vi "Convert to tiff.vi"(7 "downcast to 8-bit? (F)":bool, 8 "error in (no error)":errorcluster, 9 "source file":path, 10 "Destination directory":path, 11 "reference to path":refnum<vi>) -> (0 "error out":errorcluster)   [LabVIEW 2012]
panel:
  out "Path":path
  out "Slide":sgl(slide) scale=0.0..1.0
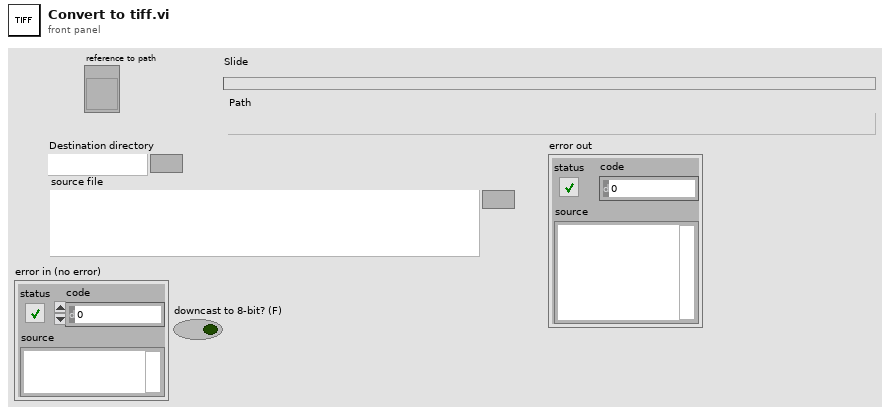
[diagram p1: front panel]
types:
  T1 = typedef "Image Type" = u32
  T2 = typedef "IMAQ Image.ctl" = refnum<image>
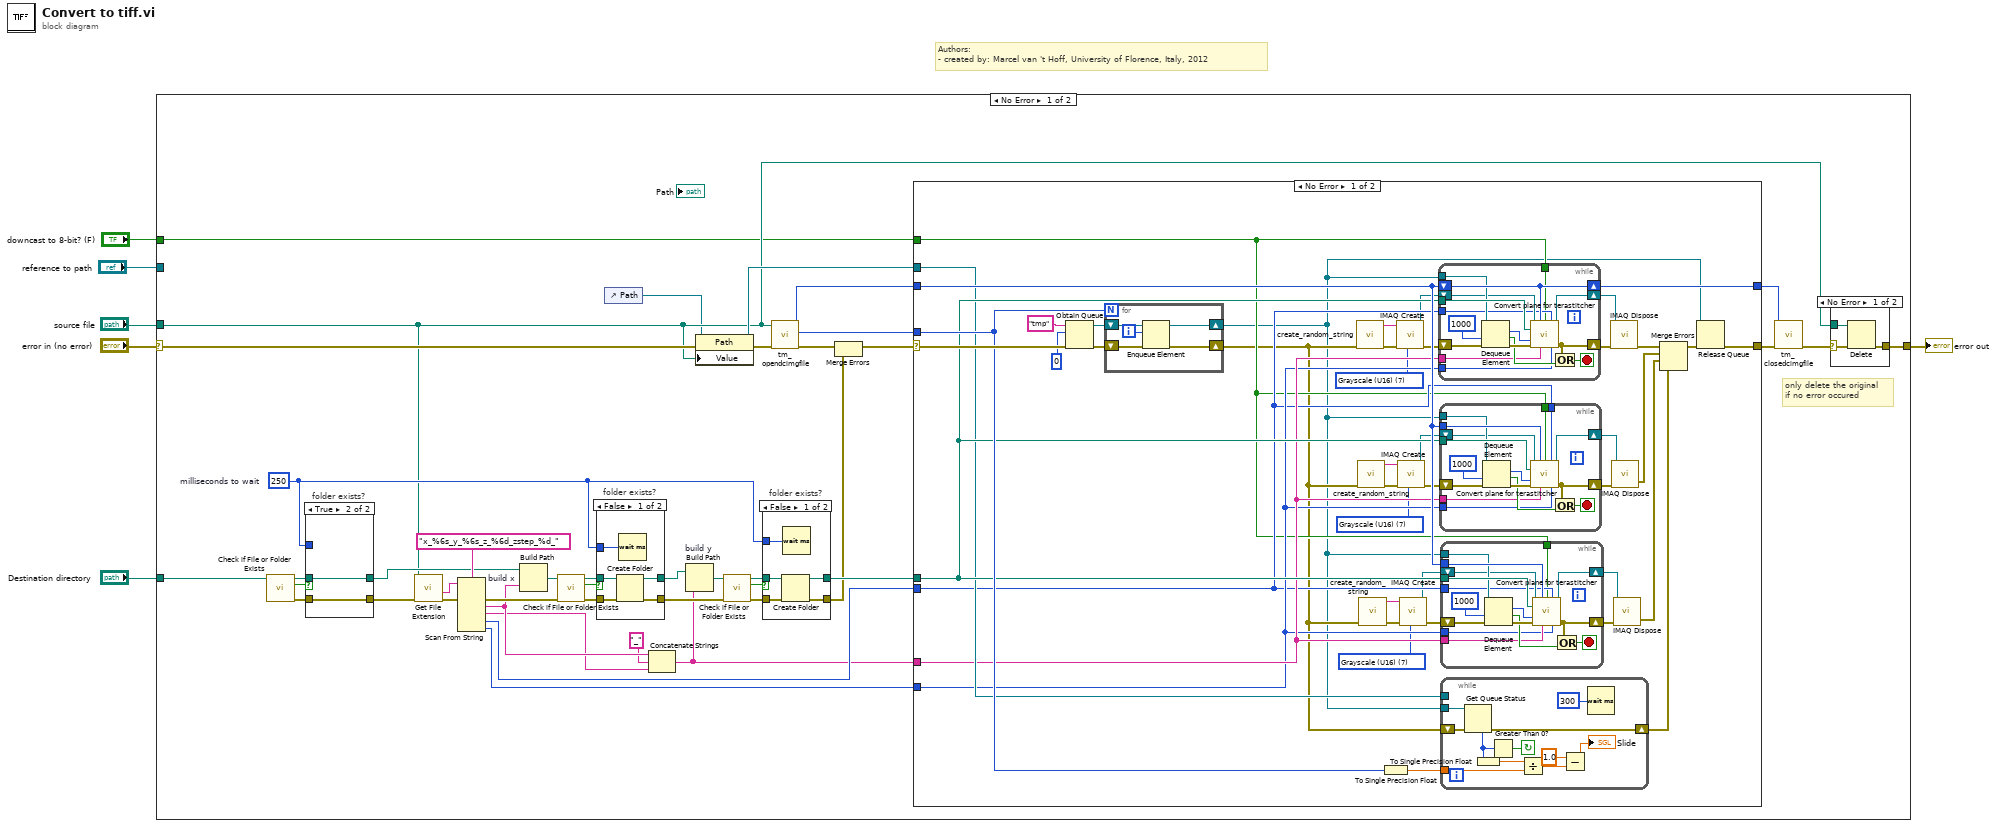
[diagram p0: block diagram]
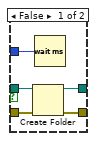
[diagram p5: hidden frame]
diagram:
  # "Authors: \n- created by: Marcel van 't Hoff, University of Florence, Italy, 2012"
  n1 = case shown="No Error" "error in (no error)" {
    selector: "error in (no error)" -> [w49 w185]
    tunnel: [w11 w185] -> w3
    tunnel: "source file" -> [w10 _]
    tunnel: "Destination directory" -> [w43 _]
    tunnel: "reference to path" -> [_ _]
    tunnel: "downcast to 8-bit? (F)" -> [w9 _]
    frame No Error {
      w12 = u32 250  # milliseconds to wait
      # "only delete the original\nif no error occured"
      n2 = call <vilib>:"Check if File or Folder Exists.vi"("path"=w43) -> ("error out"=w40:errorcluster, "file or folder exists?"=w41:bool, "dup path"=w42:path)  [unwired: 8 in]
      n3 = case "folder exists?" shown="True" w41 {
        tunnel: [w72 w74] -> w22
        tunnel: w42 -> [w71 w74]
        tunnel: w40 -> [w70 w73]
        tunnel: [w69 w73] -> w35
        tunnel: w12 -> [w68 _]
        frame False {
          n4 = Create Folder(path (use dialog)=w71, error in=w70) -> (created path=w72:path, error out=w69:errorcluster)  [unwired: 1 in, 1 out]
          n5 = Wait (ms)(milliseconds to wait=w68) -> ()  [unwired: 1 out]
        }
        frame True {
        }
      }
      n6 = call <vilib>:"Get File Extension.vi"("error in (no error)"=w35, "file"=w10) -> ("error out"=w36:errorcluster, "filename without extension"=w37:string)  [unwired: 6 in, 2 out]
      n7 = Scan From String(format string="x_%6s_y_%6s_z_%6d_zstep_%d_", input string=w37, error in=w36) -> (error out=w31:errorcluster, output 1=w21:string, output 2=w19:string, output 3=w17:i32, output 4=w18:i32)  [unwired: 5 in, 2 out]
      n8 = Build Path "build x"(base path=w22, name or relative path=w21) -> (appended path=w30:path)
      n9 = call <vilib>:"Check if File or Folder Exists.vi"("error in (no error)"=w31, "path"=w30) -> ("error out"=w34:errorcluster, "file or folder exists?"=w33:bool, "dup path"=w32:path)  [unwired: 7 in]
      n10 = case "folder exists?" shown="False" w33 {
        tunnel: [w65 w67] -> w25
        tunnel: w32 -> [w64 w67]
        tunnel: w34 -> [w63 w66]
        tunnel: [w62 w66] -> w24
        tunnel: w12 -> [w61 _]
        frame False {
          n11 = Create Folder(path (use dialog)=w64, error in=w63) -> (created path=w65:path, error out=w62:errorcluster)  [unwired: 1 in, 1 out]
          n12 = Wait (ms)(milliseconds to wait=w61) -> ()  [unwired: 1 out]
        }
        frame True {
        }
      }
      n13 = control-ref of="Path"() -> (w8:refnum<vi>)
      n14 = Concatenate Strings(w21, "_" ("string"), w19) -> (w13:string)
      n15 = Build Path "build y"(base path=w25, name or relative path=w13) -> (appended path=w29:path)
      n16 = property class="Path"(reference=w8, error in=w49, "Value"=w10) -> (reference out=w39:refnum<vi>, error out=w44:errorcluster)
      n17 = call <vilib>:"Check if File or Folder Exists.vi"("error in (no error)"=w24, "path"=w29) -> ("error out"=w26:errorcluster, "file or folder exists?"=w27:bool, "dup path"=w28:path)  [unwired: 7 in]
      n18 = case "folder exists?" shown="False" w27 {
        tunnel: [w58 w60] -> w23
        tunnel: w28 -> [w57 w60]
        tunnel: w26 -> [w56 w59]
        tunnel: [w55 w59] -> w16
        tunnel: w12 -> [w54 _]
        frame False {
          n19 = Create Folder(path (use dialog)=w57, error in=w56) -> (created path=w58:path, error out=w55:errorcluster)  [unwired: 1 in, 1 out]
          n20 = Wait (ms)(milliseconds to wait=w54) -> ()  [unwired: 1 out]
        }
        frame True {
        }
      }
      n21 = call <userlib>:"tm_opendcimgfile.vi"("error in (no error)"=w44, "Path"=w10) -> ("error out"=w15:errorcluster, "Total Frames"=w48:i32, "File Handle"=w47:u32)  [unwired: 7 in]
      n22 = Merge Errors(w15, w16) -> (w14:errorcluster)
      n23 = case shown="No Error" w14 {
        selector: w14 -> [w118 w184]
        tunnel: w47 -> [w114 w183]
        tunnel: [w116 w184] -> w45
        tunnel: w48 -> [w115 _]
        tunnel: w23 -> [w113 _]
        tunnel: w39 -> [w112 _]
        tunnel: [w117 w183] -> w46
        tunnel: w13 -> [w111 _]
        tunnel: w18 -> [w110 _]
        tunnel: w17 -> [w109 _]
        tunnel: w9 -> [w108 _]
        frame No Error {
          w88 = T1 7 items=["Grayscale (U8)", "Grayscale (I16)", "Grayscale (SGL)", "Complex (CSG)", "RGB (U32)", "HSL (U32)", "RGB (U64)", "Grayscale (U16)"] ("Image Type")
          w100 = T1 7 items=["Grayscale (U8)", "Grayscale (I16)", "Grayscale (SGL)", "Complex (CSG)", "RGB (U32)", "HSL (U32)", "RGB (U64)", "Grayscale (U16)"] ("Image Type")
          w103 = T1 7 items=["Grayscale (U8)", "Grayscale (I16)", "Grayscale (SGL)", "Complex (CSG)", "RGB (U32)", "HSL (U32)", "RGB (U64)", "Grayscale (U16)"] ("Image Type")
          n24 = Obtain Queue(name (unnamed)="tmp", element data type=0, error in (no error)=w118) -> (queue out=w83:refnum<queue>, error out=w86:errorcluster)  [unwired: 2 in, 1 out]
          n25 = for {
            N: w115 -> [_]
            shift-right: [w131] -> w82
            shift-left: w86 -> [w134]
            shift-right: [w130] -> w75
            shift-left: w83 -> [w133]
            i -> [w132]
            n26 = Enqueue Element(queue=w133, element=w132, error in (no error)=w134) -> (queue out=w130:refnum<queue>, error out=w131:errorcluster)  [unwired: 1 in, 1 out]
          }
          n27 = call "create_random_string.vi"("error in (no error)"=w82) -> ("error out"=w105:errorcluster, "random string"=w104:string)  [unwired: 9 in]
          n28 = call "create_random_string.vi"("error in (no error)"=w82) -> ("error out"=w98:errorcluster, "random string"=w99:string)  [unwired: 9 in]
          n29 = call "create_random_string.vi"("error in (no error)"=w82) -> ("error out"=w90:errorcluster, "random string"=w89:string)  [unwired: 9 in]
          n30 = To Single Precision Float(number=w115) -> (single precision float=w81:sgl)
          n31 = call "IMAQ Create"("Image Name"=w104, "Image Type"=w103, "error in (no error)"=w105) -> ("New Image"=w106:T2, "error out"=w102:errorcluster)  [unwired: 2 in]
          n32 = call "IMAQ Create"("Image Name"=w99, "Image Type"=w100, "error in (no error)"=w98) -> ("New Image"=w97:T2, "error out"=w101:errorcluster)  [unwired: 2 in]
          n33 = call "IMAQ Create"("Image Name"=w89, "Image Type"=w88, "error in (no error)"=w90) -> ("New Image"=w91:T2, "error out"=w87:errorcluster)  [unwired: 2 in]
          n34 = while {
            tunnel: w113 -> [w182]
            shift-right: [w173] -> w95
            shift-left: w102 -> [w178]
            shift-right: [w181] -> w107
            shift-left: w106 -> [w176]
            shift-right: [w180] -> w117
            shift-left: w114 -> [w180]
            tunnel: w75 -> [w179]
            tunnel: w111 -> [w170]
            tunnel: w110 -> [w169]
            tunnel: w109 -> [w168]
            tunnel: w108 -> [w167]
            stop <- w171 stop-if-true
            n35 = Dequeue Element(queue=w179, timeout in ms (-1)=1000, error in (no error)=w178) -> (element=w177:i32, timed out?=w172:bool, error out=w174:errorcluster)  [unwired: 1 out]
            n36 = call "Convert plane for terastitcher.vi"("Image in"=w176, "File Handle"=w180, "downcast to 8-bit? (F)"=w167, "z start position"=w168, "file in"=w182, "Frame Index"=w177, "error in (no error)"=w174, "basepath name"=w170, "z step size"=w169) -> ("Image out"=w181:T2, "error out"=w173:errorcluster)  [unwired: 5 in]
            n37 = Or(x=w173, y=w172) -> (x .or. y?=w171:bool)
          }
          n38 = while {
            tunnel: w113 -> [w166]
            shift-right: [w155] -> w94
            shift-left: w101 -> [w162]
            shift-right: [w165] -> w96
            shift-left: w97 -> [w159]
            tunnel: w75 -> [w163]
            tunnel: w114 -> [w164]
            tunnel: w111 -> [w154]
            tunnel: w110 -> [w153]
            tunnel: w109 -> [w152]
            tunnel: w108 -> [w151]
            stop <- w156 stop-if-true
            n39 = Dequeue Element(queue=w163, timeout in ms (-1)=1000, error in (no error)=w162) -> (element=w160:i32, timed out?=w157:bool, error out=w161:errorcluster)  [unwired: 1 out]
            n40 = call "Convert plane for terastitcher.vi"("Image in"=w159, "File Handle"=w164, "downcast to 8-bit? (F)"=w151, "z start position"=w152, "file in"=w166, "Frame Index"=w160, "error in (no error)"=w161, "basepath name"=w154, "z step size"=w153) -> ("Image out"=w165:T2, "error out"=w155:errorcluster)  [unwired: 5 in]
            n41 = Or(x=w155, y=w157) -> (x .or. y?=w156:bool)
          }
          n42 = while {
            tunnel: w113 -> [w150]
            shift-right: [w139] -> w93
            shift-left: w87 -> [w146]
            shift-right: [w149] -> w92
            shift-left: w91 -> [w143]
            tunnel: w75 -> [w147]
            tunnel: w114 -> [w148]
            tunnel: w111 -> [w138]
            tunnel: w110 -> [w137]
            tunnel: w109 -> [w136]
            tunnel: w108 -> [w135]
            stop <- w140 stop-if-true
            n43 = Dequeue Element(queue=w147, timeout in ms (-1)=1000, error in (no error)=w146) -> (element=w144:i32, timed out?=w141:bool, error out=w145:errorcluster)  [unwired: 1 out]
            n44 = call "Convert plane for terastitcher.vi"("Image in"=w143, "File Handle"=w148, "downcast to 8-bit? (F)"=w135, "z start position"=w136, "file in"=w150, "Frame Index"=w144, "error in (no error)"=w145, "basepath name"=w138, "z step size"=w137) -> ("Image out"=w149:T2, "error out"=w139:errorcluster)  [unwired: 5 in]
            n45 = Or(x=w139, y=w141) -> (x .or. y?=w140:bool)
          }
          n46 = while {
            tunnel: w75 -> [w129]
            tunnel: w112 -> [_]
            shift-right: [w120] -> w78
            shift-left: w82 -> [w127]
            tunnel: w81 -> [w125]
            stop <- w128 continue-if-true
            n47 = Get Queue Status(queue=w129, error in (no error)=w127) -> (error out=w120:errorcluster, # elements in queue=w126:i32)  [unwired: 1 in, 6 out]
            n48 = To Single Precision Float(number=w126) -> (single precision float=w124:sgl)
            n49 = Greater Than 0?(x=w126) -> (x > 0?=w128:bool)
            n50 = Divide(x=w124, y=w125) -> (x/y=w122:sgl)
            n51 = Subtract(x=sgl 1.0, y=w122) -> (x-y=→"Slide":sgl)
            n52 = Wait (ms)(milliseconds to wait=u32 300) -> ()  [unwired: 1 out]
          }
          n53 = call "IMAQ Dispose"("Image"=w107, "error in (no error)"=w95) -> ("error out"=w77:errorcluster)  [unwired: 4 in]
          n54 = call "IMAQ Dispose"("Image"=w96, "error in (no error)"=w94) -> ("error out"=w80:errorcluster)  [unwired: 4 in]
          n55 = call "IMAQ Dispose"("Image"=w92, "error in (no error)"=w93) -> ("error out"=w79:errorcluster)  [unwired: 4 in]
          n56 = Merge Errors(w77, w80, w79, w78) -> (w76:errorcluster)
          n57 = Release Queue(queue=w75, error in (no error)=w76) -> (error out=w116:errorcluster)  [unwired: 1 in, 2 out]
        }
        frame Error {
        }
      }
      n58 = call <userlib>:"tm_closedcimgfile.vi"("error in (no error)"=w45, "File Handle"=w46) -> ("error out"=w7:errorcluster)  [unwired: 9 in]
      n59 = case shown="No Error" w7 {
        selector: w7 -> [w50 w53]
        tunnel: [w52 w53] -> w11
        tunnel: w10 -> [w51 _]
        frame No Error {
          n60 = Delete(path (use dialog)=w51, error in=w50) -> (error out=w52:errorcluster)  [unwired: 3 in, 2 out]
        }
        frame Error {
        }
      }
    }
    frame Error {
    }
  }
  "error out" <- w3
